vi "_Buffer_To_AllElements.vi"(10 "count (-1: all)":i32=-1, 11 "Buffer":refnum<class "VariantBuffer.lvclass">) -> (3 "elements":variant[](array[variant]))   [LabVIEW 2013, in "VariantBuffer.lvclass"]
uses:
  VariantBuffer.lvclass
  VariantBuffer.lvclass/VariantBuffer.ctl
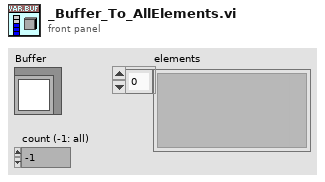
[diagram p1: front panel]
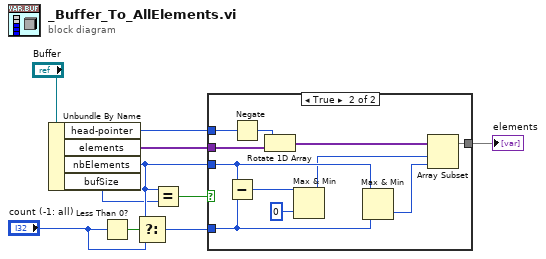
[diagram p0: block diagram]
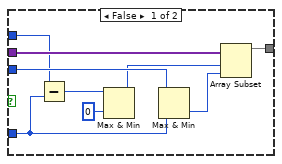
[diagram p2: hidden frame]
diagram:
  n1 = Unbundle By Name("Buffer") -> ("head-pointer"=w5:i32, "elements"=w2:variant[], "nbElements"=w9:i32, "bufSize"=w6:i32)
  n2 = Less Than 0?(x="count (-1: all)") -> (x < 0?=w7:bool)
  n3 = Select(t=w9, s=w7, f="count (-1: all)") -> (s? t:f=w8:i32)
  n4 = Equal?(x=w9, y=w6) -> (x = y?=w1:bool)
  n5 = case shown="True" w1 {
    tunnel: w2 -> [w17 w30]
    tunnel: [w19 w28] -> w4
    tunnel: w8 -> [w13 w24]
    tunnel: w5 -> [w11 w22]
    tunnel: w9 -> [w14 w21]
    frame False {
      n6 = Subtract(x=w11, y=w13) -> (x-y=w16:i32)
      n7 = Max & Min(x=w16, y=0) -> (max(x,y)=w12:i32)  [unwired: 1 out]
      n8 = Max & Min(x=w14, y=w13) -> (min(x,y)=w18:i32)  [unwired: 1 out]
      n9 = Array Subset(array=w17, index=w12, length=w18) -> (w19:variant[])
    }
    frame True {
      n10 = Subtract(x=w21, y=w24) -> (x-y=w26:i32)
      n11 = Negate(x=w22) -> (-x=w27:i32)
      n12 = Rotate 1D Array(1:w30, 2:w27) -> (0:w29:variant[])
      n13 = Max & Min(x=w26, y=0) -> (max(x,y)=w20:i32)  [unwired: 1 out]
      n14 = Max & Min(x=w21, y=w24) -> (min(x,y)=w23:i32)  [unwired: 1 out]
      n15 = Array Subset(array=w29, index=w20, length=w23) -> (w28:variant[])
    }
  }
  "elements" <- w4
